vi "User Event Abort.vi"(8 "error in":errorcluster, 11 "Action":T1) -> (0 "error out":errorcluster, 3 "user event out":refnum<user-event>)   [LabVIEW 2025]
doc: "This VI creates, provides access to and destroys the user event abort all."
uses:
  Controls/UE Abort Action.ctl
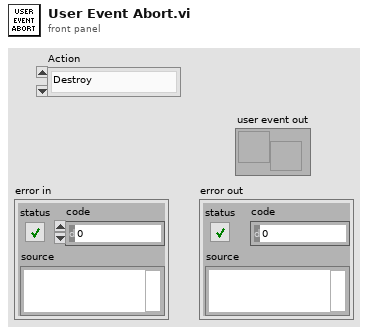
[diagram p1: front panel]
types:
  T1 = typedef "UE Abort Action.ctl" = enum16{"Destroy", "Get", "Create"}
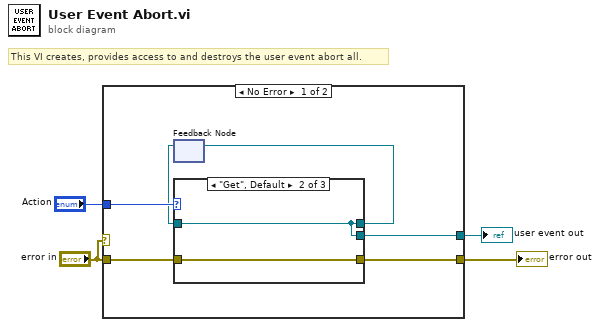
[diagram p0: block diagram]
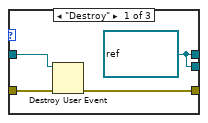
[diagram p2: hidden frame]
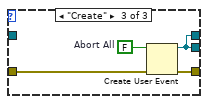
[diagram p3: hidden frame]
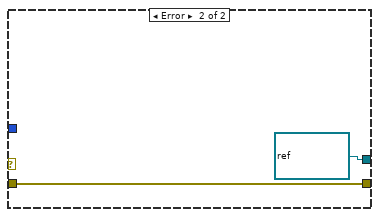
[diagram p4: hidden frame]
diagram:
  # "This VI creates, provides access to and destroys the user event abort all."
  n1 = case shown="No Error" "error in" {
    tunnel: "error in" -> [w10 w22]
    tunnel: "Action" -> [w9 _]
    tunnel: [w8 w22] -> w3
    tunnel: [w5 refnum<user-event> refnum ("Abort All")] -> w2
    frame No Error {
      n2 = feedback #1() -> (w6:refnum<user-event>)  [unwired: 1 in]
      n3 = case shown="\"Get\", Default" w9 {
        tunnel: w10 -> [w14 w15 w20]
        tunnel: [w13 w15 w19] -> w8
        tunnel: [w11 w16 w17] -> w7
        tunnel: w6 -> [w12 w16 _]
        tunnel: [w11 w16 w17] -> w5
        frame "Destroy" {
          w11 = refnum<user-event> refnum ("user event")
          n4 = Destroy User Event(user event=w12, error in=w14) -> (error out=w13:errorcluster)
        }
        frame "Get", Default {
        }
        frame "Create" {
          w18 = FALSE  # Abort All
          n5 = Create User Event(user event datatype=w18, error in=w20) -> (user event=w17:refnum<user-event>, error out=w19:errorcluster)
        }
      }
      n6 = feedback-in #1(w7) -> ()
    }
    frame Error {
    }
  }
  "error out" <- w3
  "user event out" <- w2
